vi "OSICS_Get_Wavelength.vi"(7 "OSICS slot":i32=1 min=1 max=8 step=1, 8 "error in":errorcluster, 10 "WL/F unit (False:NM)":bool, 11 "VISA IN":refnum<visa-resource-name>) -> (0 "error out":errorcluster, 2 "WL/Frequency Value":dbl format="%.3f", 3 "VISA OUT":refnum<visa-resource-name>, 5 "ERR":i32)   [LabVIEW 2014, in "OSICS_LIB.lvlib"]
doc: "This Vi reads the wavelength or Frequency settings of OSICS modules depending on the input Wavelength/Frequency unit.\nModules: DFB, ECL, SLED, T100, TLS-50, TLS-AG."
uses:
  OSICS_LIB.lvlib
panel:
  # "Basic Function to read the wavelength / Frequency \nof the OSICS"
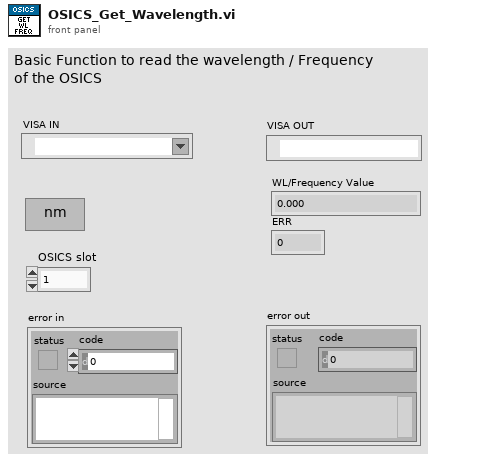
[diagram p1: front panel]
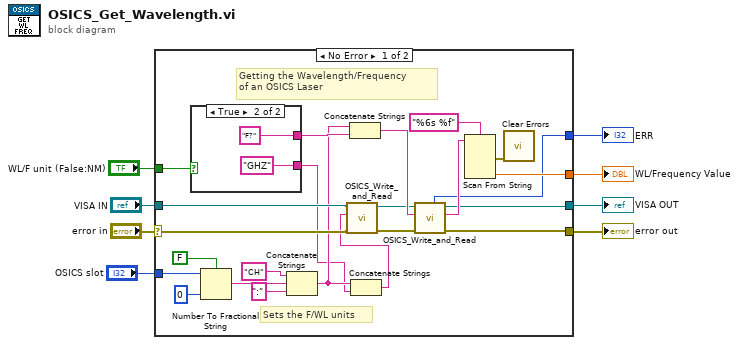
[diagram p0: block diagram]
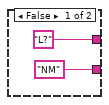
[diagram p2: hidden frame]
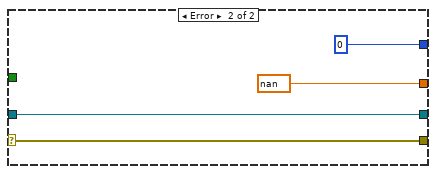
[diagram p3: hidden frame]
diagram:
  n1 = case shown="No Error" "error in" {
    selector: "error in" -> [w14 w38]
    tunnel: "WL/F unit (False:NM)" -> [w31 _]
    tunnel: "VISA IN" -> [w13 w39]
    tunnel: [w19 w39] -> w7
    tunnel: [w20 w38] -> w6
    tunnel: [w29 nan] -> w4
    tunnel: [w18 0 ("ERR")] -> w2
    tunnel: "OSICS slot" -> [w26 _]
    frame No Error {
      # "Sets the F/WL units"
      # "Getting the Wavelength/Frequency\nof an OSICS Laser"
      n2 = case shown="True" w31 {
        tunnel: ["L?" "F?"] -> w17
        tunnel: ["NM" "GHZ"] -> w10
        frame False {
        }
        frame True {
        }
      }
      n3 = Number To Fractional String(use system decimal point (T)=FALSE, number=w26, precision (6)=i16 0) -> (F-format string=w22:string)  [unwired: 1 in]
      n4 = Concatenate Strings("CH" ("string"), w22, ":" ("string")) -> (w11:string)
      n5 = Concatenate Strings(w11, w17) -> (w16:string)
      n6 = Concatenate Strings(w11, w10) -> (w9:string)
      n7 = call "OSICS_Write_and_Read.vi"("error in (no error)"=w14, "String to Send"=w9, "VISA IN"=w13) -> ("error out"=w15:errorcluster, "VISA OUT"=w12:refnum<visa-resource-name>)  [unwired: 5 in, 2 out]
      n8 = call "OSICS_Write_and_Read.vi"("error in (no error)"=w15, "String to Send"=w16, "VISA IN"=w12) -> ("error out"=w20:errorcluster, "Message Available"=w28:string, "VISA OUT"=w19:refnum<visa-resource-name>, "ERR"=w18:i32)  [unwired: 5 in]
      n9 = Scan From String(format string="%6s %f", input string=w28) -> (error out=w27:errorcluster, output 2=w29:dbl)  [unwired: 5 in, 2 out]
      n10 = call <vilib>:"Clear Errors.vi"("error in (no error)"=w27) -> ()  [unwired: 5 in, 2 out]
    }
    frame Error {
    }
  }
  "error out" <- w6
  "VISA OUT" <- w7
  "WL/Frequency Value" <- w4
  "ERR" <- w2
